vi "Ch_Selector.vi"(0 "Devices":string[](array[string])) -> (1 "Ch_type_index":i32[](array[numeric]), 2 "Device_Present?":bool[](array[boolean]))   [LabVIEW 2013]
panel:
  out "output string":string
  # "Type Index\n0 = TEMP\n1 = HTR\n2 = AUX\n3 = LVL\n4 = PRES\n5 = FLW\n6 = Empty"
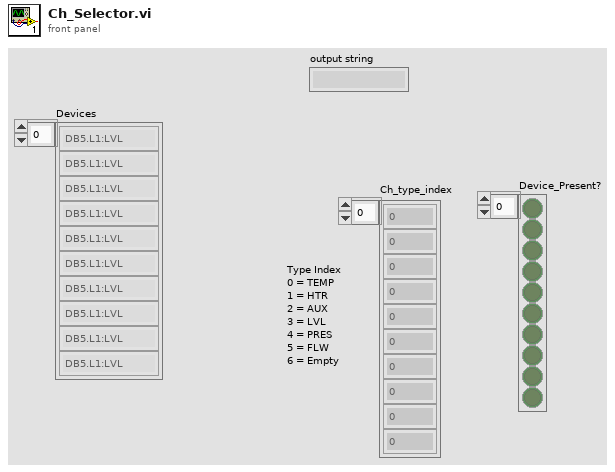
[diagram p1: front panel]
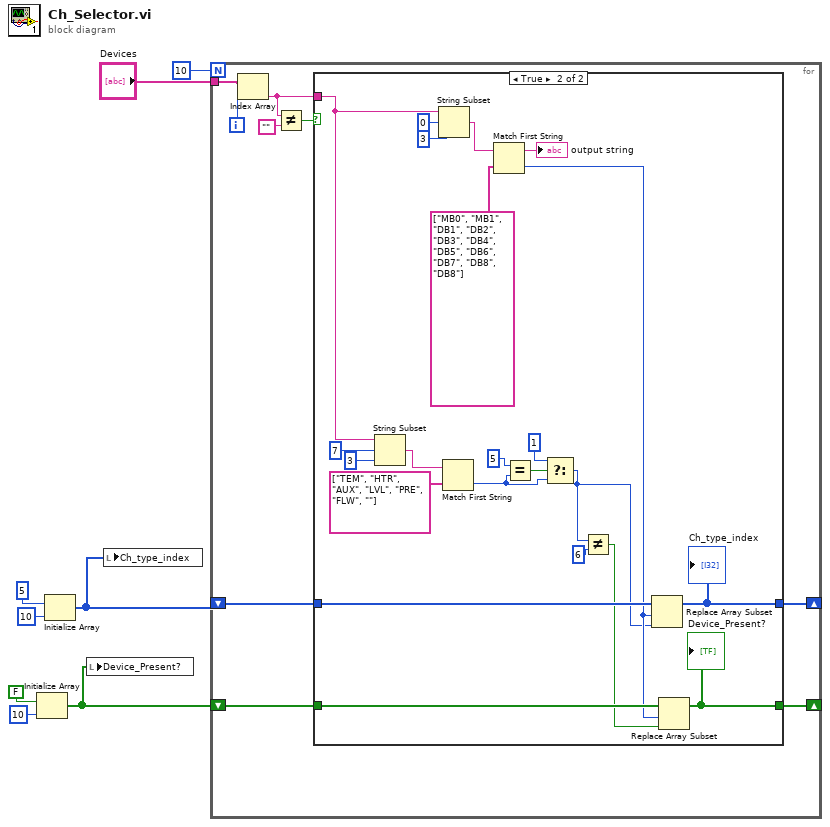
[diagram p0: block diagram]
diagram:
  n1 = Initialize Array(FALSE, 10 ("dimension size")) -> (w1:bool[])
  n2 = Initialize Array(5 ("dimension size"), 10 ("dimension size")) -> (w2:i32[])
  n3 = local write "Device_Present?"(w1) -> ()
  n4 = local write "Ch_type_index"(w2) -> ()
  n5 = for {
    N: 10 -> [_]
    tunnel: "Devices" -> [w16]
    shift-right: [w14] -> _
    shift-left: w2 -> [w15]
    shift-right: [w12] -> _
    shift-left: w1 -> [w13]
    i -> [w17]
    n6 = Index Array(array=w16, index=w17) -> (element=w10:string)
    n7 = Not Equal?(x=w10, y="") -> (x != y?=w9:bool)
    n8 = case shown="True" w9 {
      tunnel: w15 -> [w19 w31]
      tunnel: [w19 w30] -> w14
      tunnel: w13 -> [w18 w29]
      tunnel: [w18 w27] -> w12
      tunnel: w10 -> [_ w25]
      frame False {
      }
      frame True {
        n9 = String Subset(string=w25, offset (0)=7, length (rest)=3 ("length (rest)")) -> (substring=w39:string)
        n10 = String Subset(string=w25, offset (0)=0, length (rest)=3 ("length (rest)")) -> (substring=w34:string)
        n11 = Match First String(2:string[] ["TEM", "HTR", "AUX", "LVL", "PRE", "FLW", ""] ("string array"), 3:w39) -> (0:w22:i32)  [unwired: 1 out]
        n12 = Match First String(2:string[] ["MB0", "MB1", "DB1", "DB2", "DB3", "DB4", "DB5", "DB6", "DB7", "DB8", "DB8"], 3:w34) -> (0:w28:i32, 1:→"output string":string)
        n13 = Equal?(x=5 ("y"), y=w22) -> (x = y?=w24:bool)
        n14 = Select(t=1 ("y"), s=w24, f=w22) -> (s? t:f=w21:i32)
        n15 = Not Equal?(x=w21, y=6) -> (x != y?=w26:bool)
        n16 = Replace Array Subset(array=w31, new element=w21, index=w28) -> (w30:i32[])
        "Ch_type_index" <- w30
        n17 = Replace Array Subset(array=w29, new element=w26, index=w28) -> (w27:bool[])
        "Device_Present?" <- w27
      }
    }
  }
